vi "Send Message.vi"(0 "message queue in":T3, 1 "receiver port":u16, 2 "force UDP port":bool, 5 "message":T1, 9 "timeout (-1 ms)":i32=-1, 11 "error in":errorcluster) -> (4 "message queue out":T3, 10 "timed out?":bool, 15 "error out":errorcluster)   [LabVIEW 2013, in "AMC.lvlib"]
doc: "Adds a message to:\n- the local queue passed in by reference if \"receiver host\" and \"receiver process\" are left undefined\n- another message queue on the local target if \"receiver host\" is undefined, but \"receiver process\" is specified\n- the message dispatch queue in another application instance if the receiver host and process are specified.\n\nIf \"receiver port\" is undefined, this VI will attempt to use the default UDP port or the port stored in the send-to string. If the forced boolean is set, it uses the old behavior of using the input or default udp port\n\n\nIf \"priority message\" is True, the message will be added to the front of the message queue.\n\nIf \"acknowledge message\" is True and the message is sent to another application instance, the receiver will send a reply message with the name format of \"AMC_Ack\" and a value of <name>. If \"message queue in\" is undefined, no acknowledge message will be sent."
uses:
  AMC.lvlib
  Message Queue.ctl
  Message.ctl
  <vilib>/NI/Tools/Keyed Array/KeyedArray.ctl
  <vilib>/NI/Tools/Keyed Array/Tools_KeyedArray.lvlib
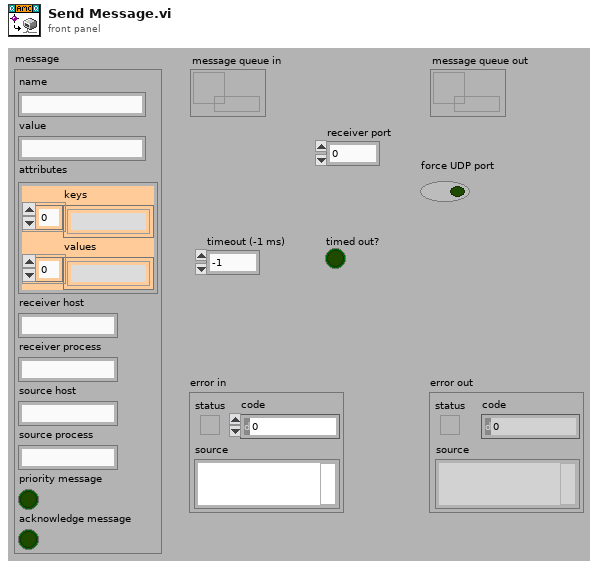
[diagram p1: front panel]
types:
  T1 = typedef "AMC.lvlib/Message.ctl" = cluster{"name":string, "value":string, "attributes":T2, "receiver host":string, "receiver process":string, "source host":string, "source process":string, "priority message":bool, "acknowledge message":bool}
  T2 = typedef "Tools_KeyedArray.lvlib/KeyedArray.ctl" = cluster{"keys":string[], "values":string[]}
  T3 = typedef "AMC.lvlib/Message Queue.ctl" = refnum<queue>
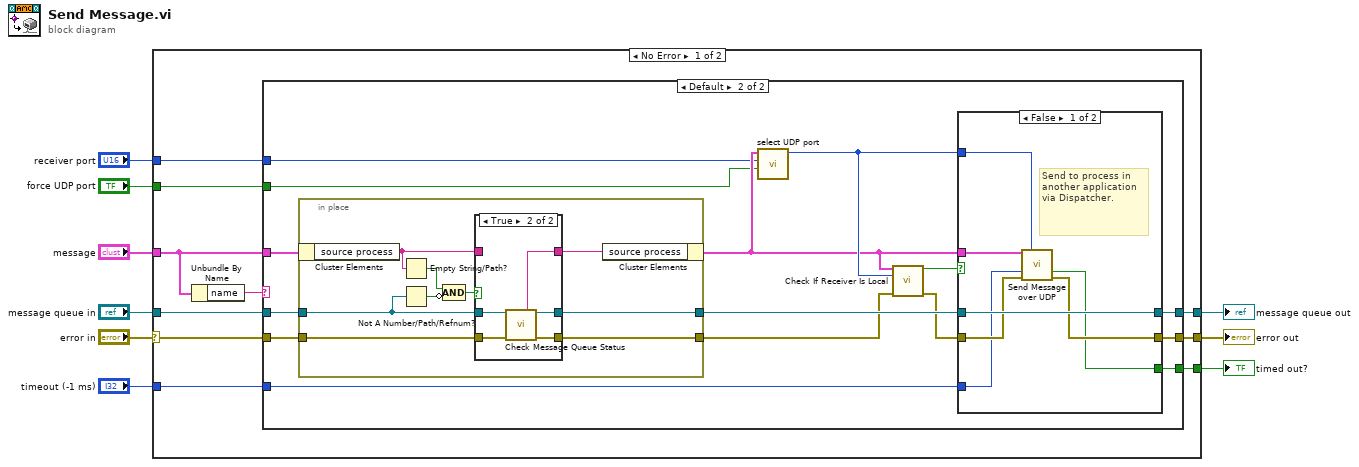
[diagram p0: block diagram]
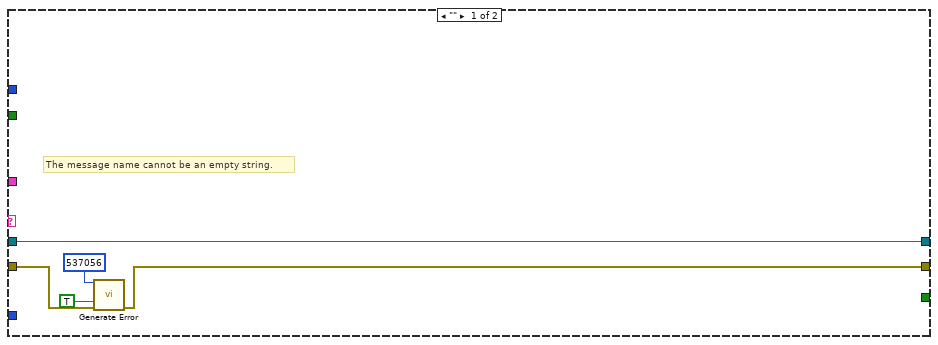
[diagram p2: hidden frame]
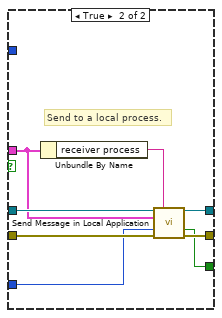
[diagram p4: hidden frame]
diagram:
  n1 = case shown="No Error" "error in" {
    selector: "error in" -> [w16 w72]
    tunnel: [w19 w72] -> w9
    tunnel: "message queue in" -> [w17 w73]
    tunnel: [w18 w73] -> w7
    tunnel: "message" -> [w12 _]
    tunnel: "timeout (-1 ms)" -> [w15 _]
    tunnel: [w14 _] -> w3
    tunnel: "receiver port" -> [w13 _]
    tunnel: "force UDP port" -> [w10 _]
    frame No Error {
      n2 = Unbundle By Name(w12) -> ("name"=w11:string)
      n3 = case shown="Default" w11 {
        tunnel: [w21 w39] -> w19
        tunnel: [w24 w38] -> w18
        tunnel: w17 -> [w24 w37]
        tunnel: w16 -> [w22 w36]
        tunnel: w15 -> [_ w34]
        tunnel: [_ w33] -> w14
        tunnel: w13 -> [_ w26]
        tunnel: w12 -> [_ w29]
        tunnel: w10 -> [_ w25]
        frame "" {
          # "The message name cannot be an empty string."
          n4 = call "Generate Error.vi"("code"=537056, "status (F)"=TRUE, "error in"=w22) -> ("error out"=w21:errorcluster)  [unwired: 12 in]
        }
        frame Default {
          n5 = in-place {
            in-place-border: w37 -> [w43]
            in-place-border: w36 -> [w48]
            in-place-border: [w47] -> w35
            in-place-border: [w46] -> w30
            n6 = in-place-cluster #1(w29) -> ("source process"=w45:string)
            n7 = Empty String/Path?(string/path=w45) -> (empty?=w41:bool)
            n8 = Not A Number/Path/Refnum?(number/path/refnum=w43) -> (NaN/Path/Refnum?=w42:bool)
            n9 = Compound Arithmetic op=AND(w41, invert w42) -> (w40:bool)
            n10 = case shown="True" w40 {
              tunnel: w43 -> [w51 w56]
              tunnel: w48 -> [w50 w55]
              tunnel: [w51 w54] -> w47
              tunnel: [w50 w53] -> w46
              tunnel: [w49 w52] -> w44
              tunnel: w45 -> [w49 _]
              frame False {
              }
              frame True {
                n11 = call "Check Message Queue Status.vi"("message queue in"=w56, "error in"=w55) -> ("message queue name"=w52:string, "message queue out"=w54:T3, "error out"=w53:errorcluster)  [unwired: 9 in, 2 out]
              }
            }
            n12 = in-place-cluster #1("source process"=w44) -> (w27:T1)
          }
          n13 = call "select UDP port.vi"("force UDP port"=w25, "receiver port (if not in target or forced, use global default)"=w26, "message"=w27) -> ("receiver port (global default)"=w28:u16)  [unwired: 8 in]
          n14 = call "Check If Receiver Is Local.vi"("message"=w27, "UDP receiver port"=w28, "error in"=w30) -> ("local receiver?"=w32:bool, "error out"=w31:errorcluster)  [unwired: 11 in]
          n15 = case shown="False" w32 {
            tunnel: w31 -> [w61 w69]
            tunnel: [w62 w68] -> w39
            tunnel: w35 -> [w63 w71]
            tunnel: [w63 w70] -> w38
            tunnel: w27 -> [w57 w65]
            tunnel: w34 -> [w60 w67]
            tunnel: [w59 w66] -> w33
            tunnel: w28 -> [w58 _]
            frame False {
              # "Send to process in another application via Dispatcher."
              n16 = call "Send Message over UDP.vi"("message"=w57, "UDP receiver port (if not found)"=w58, "timeout (25000 ms)"=w60, "error in"=w61) -> ("timed out?"=w59:bool, "error out"=w62:errorcluster)  [unwired: 9 in, 1 out]
            }
            frame True {
              # "Send to a local process."
              n17 = Unbundle By Name(w65) -> ("receiver process"=w64:string)
              n18 = call "Send Message in Local Application.vi"("message queue in"=w71, "receiver process (\"\" - local)"=w64, "message"=w65, "timeout (-1 ms)"=w67, "error in"=w69) -> ("message queue out"=w70:T3, "timed out?"=w66:bool, "error out"=w68:errorcluster)  [unwired: 8 in]
            }
          }
        }
      }
    }
    frame Error {
    }
  }
  "error out" <- w9
  "message queue out" <- w7
  "timed out?" <- w3
